vi "DataFinder Query.vi"(6 "result columns (comma list)":string, 7 "Run search type (\"\")":string, 8 "error in (no error)":errorcluster, 11 "Query Parameters":T2={"UserName"="", "Search Parameters"=[], "eSearch Type"=enum."eSearchFile", "Query Name (vbs)"="Spartan_Query.VBS", "Response queue name"="", "Logic String"=""}) -> (0 "error out":errorcluster, 1 "Results":string[][](array[string]), 2 "Items":string[][](array[string]), 3 "Item Filenames":string[](array[string]), 4 "runs":T1[](array[typedef]), 5 "Item Filepaths":string[](array[string]))   [LabVIEW 2011]
uses:
  DIAdem/lib/DIAdem Query Queue.ctl
  Datafinder Query.ctl
  eSearch Types.ctl
  DataFinder Comparisons.ctl
  www/cgi-bin/_cgi-lib/TDM_INDEX Record.ctl
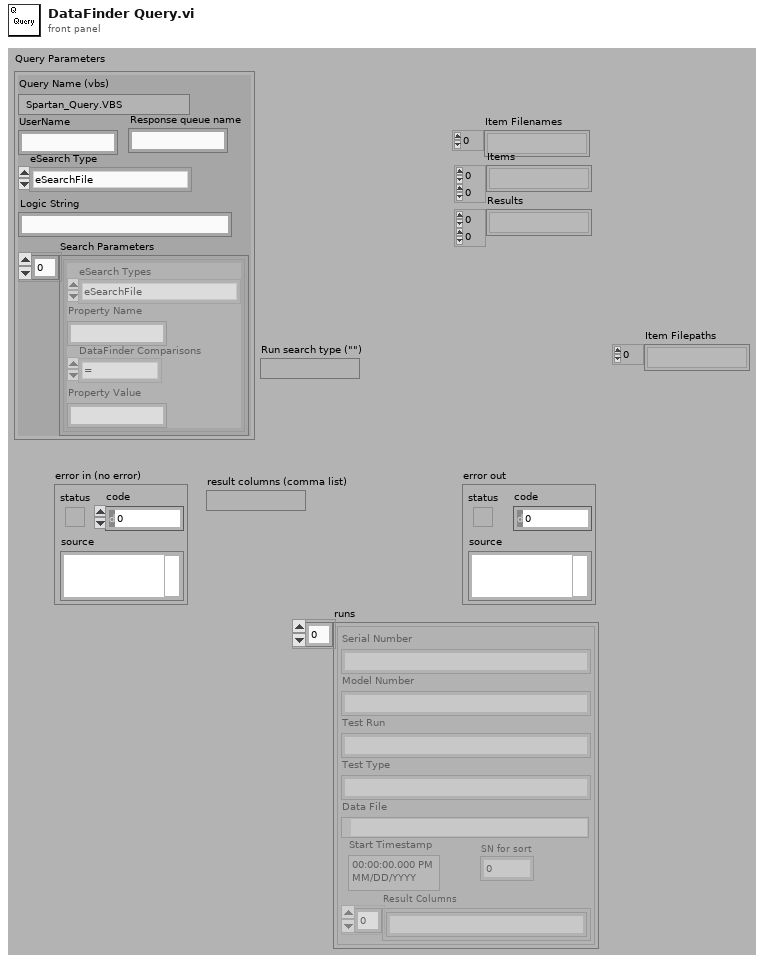
[diagram p1: front panel]
types:
  T1 = typedef "TDM_INDEX Record.ctl" = cluster{"Model Number":string, "SN for sort":i32, "Test Type":string, "Test Run":string, "Serial Number":string, "Start Timestamp":timestamp, "Data File":path, "Result Columns":string[]}
  T2 = typedef "DIAdem Query Queue.ctl" = cluster{"UserName":string, "Search Parameters":T3[], "eSearch Type":T4, "Query Name (vbs)":string, "Response queue name":string, "Logic String":string}
  T3 = typedef "Datafinder Query.ctl" = cluster{"eSearch Types":T4, "Property Name":string, "DataFinder Comparisons":T5, "Property Value":string}
  T4 = typedef "eSearch Types.ctl" = enum16{"eSearchFile", "eSearchChannelGroup", "eSearchChannel"}
  T5 = typedef "DataFinder Comparisons.ctl" = enum16{"=", "<>", "<", "<=", ">", ">="}
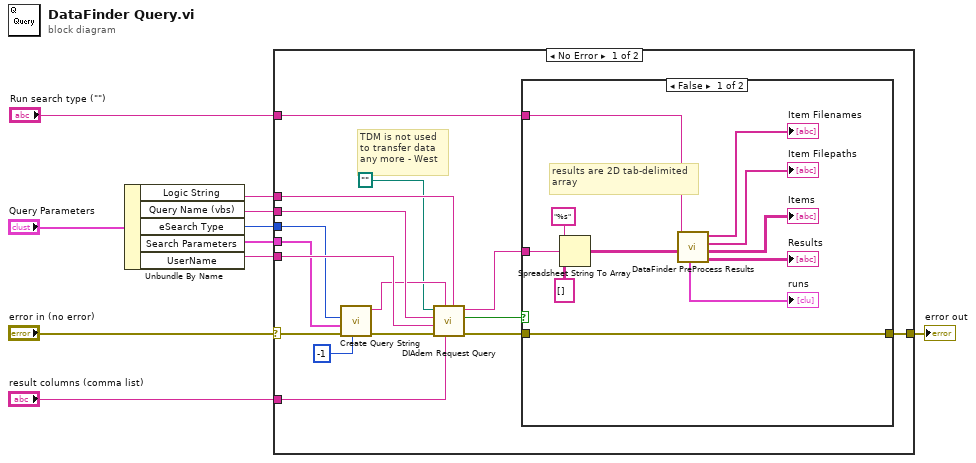
[diagram p0: block diagram]
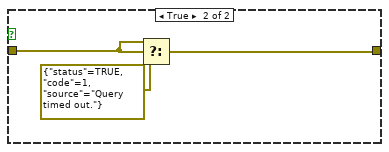
[diagram p2: hidden frame]
diagram:
  n1 = Unbundle By Name("Query Parameters") -> ("Logic String"=w3:string, "Query Name (vbs)"=w8:string, "eSearch Type"=w7:T4, "Search Parameters"=w6:T3[], "UserName"=w5:string)
  n2 = case shown="No Error" "error in (no error)" {
    selector: "error in (no error)" -> [w18 w41]
    tunnel: [w12 w41] -> w2
    tunnel: w5 -> [w25 _]
    tunnel: w6 -> [w24 _]
    tunnel: w7 -> [w23 _]
    tunnel: w8 -> [w22 _]
    tunnel: w3 -> [w20 _]
    tunnel: "result columns (comma list)" -> [w19 _]
    tunnel: "Run search type (\"\")" -> [w11 _]
    frame No Error {
      # "TDM is not used\nto transfer data\nany more - West"
      n3 = call "Create Query String.vi"("Max Results (-1 is ALL)"=-1 ("Max Results (-1 is 5000)"), "error in (no error)"=w18, "DataFinder parameters"=w24, "Return Type (ChannelGroup)"=w23) -> ("error out"=w26:errorcluster, "Query String Out"=w21:string)  [unwired: 1 in, 5 out]
      n4 = call "DIAdem Request Query.vi"("Logic String"=w20, "result columns (comma list)"=w19, "Conditions String"=w21, "error in (no error)"=w26, "Username (empty)"=w25, "Query Name"=w22, "Query TDM"=path "") -> ("error out"=w14:errorcluster, "Timed Out?"=w15:bool, "Result"=w13:string)  [unwired: 2 out]
      n5 = case shown="False" w15 {
        tunnel: w14 -> [w34 w40]
        tunnel: w13 -> [w37 _]
        tunnel: [w34 w38] -> w12
        tunnel: w11 -> [w32 _]
        frame False {
          # "results are 2D tab-delimited\narray"
          n6 = Spreadsheet String To Array(format string="%s", spreadsheet string=w37, array type (2D Dbl)=string[][] [] ("Results")) -> (array=w33:string[][])  [unwired: 1 out]
          n7 = call "DataFinder PreProcess Results.vi"("Raw Results (empty)"=w33, "RUNSELECT (\"\")"=w32) -> ("Results"=→"Results":string[][], "Items"=→"Items":string[][], "Item Filepaths"=→"Item Filepaths":string[], "Item Filenames"=→"Item Filenames":string[], "runs"=→"runs":T1[])  [unwired: 5 in]
        }
        frame True {
          n8 = Select(t=w40, s=w40, f=errorcluster {"status"=TRUE, "code"=1, "source"="Query timed out."} ("error IO")) -> (s? t:f=w38:errorcluster)
        }
      }
    }
    frame Error {
      # "This query is dead"
    }
  }
  "error out" <- w2
